vi "190627_FreCTO.vi"() -> ()   [LabVIEW 2019]
uses:
  <vilib>/rvi/interface/nirviReadWriteControl/nirviReadWriteControl.xnode
  <vilib>/rvi/interface/Simulation/niFpgaSimulationCallBeginRW.vi
  <vilib>/rvi/errors/niLvFpgaAdjustHostInterfaceError.vi
  <vilib>/rvi/interface/nirviMethod/nirviMethod.xnode
  <vilib>/FPGAPlugInAG/Dynamic/niLvFpga_Reset_Dynamic.vi
  <vilib>/FPGAPlugInAG/Dynamic/niLvFpga_Run_Dynamic.vi
  <vilib>/rvi/interface/nirviCloseFPGA/nirviCloseFPGA.xnode
  <vilib>/Platform/TimedLoop/XDataNode/XDataNode.xnode
  <vilib>/Platform/TimedLoop/XDataNode/nitl_modes.ctl
  <vilib>/Platform/TimedLoop/XDataNode/XDNodeRunTimeDep.lvlib
  <vilib>/Platform/TimedLoop/XDataNode/wakeup.ctl
  <vilib>/Platform/TimedLoop/XDataNode/timing_clust.ctl
  <vilib>/rvi/interface/nirviOpenFPGA/nirviOpenFPGA.xnode
  <vilib>/Utility/Variable/NI_VariableUtilities.lvlib
  FPGA_TwoAxisEncoder_revised.vi
  <vilib>/FPGAPlugInAG/Dynamic/niLvFpga_Close_Dynamic.vi
panel:
  in  "X_Type":string(combo)="Notch15"
  in  "X_pole":string(combo)="4352"
  in  "Z_Type":string(combo)="Notch15"
  in  "Z_pole":string(combo)="4952"
  out "Time Slots (sec)":dbl[](array[numeric])
  out "All times (sec)":dbl
  out "one period  length":i32
  out "one period start time":i32
  in  "HOST Sample Rate (Hz)":i32=1000
  in  "LOAD":bool
  out "(LS) RMS X (one) (um)":dbl format="%0.4f"
  out "(LS) MAX ERROR X (um)":dbl format="%0.4f"
  out "(LS) RMS ERROR X (um)":dbl format="%0.4f"
  out "(En) RMS X (one) (um)":dbl format="%0.4f"
  out "(LS) RMS Z (one) (um)":dbl format="%0.4f"
  out "(LS) MAX ERROR Z (um)":dbl format="%0.4f"
  out "(LS) RMS ERROR Z (um)":dbl format="%0.4f"
  out "CMD X (rpm)":dbl[](graph)
  out "Linear Scale Position X (mm)":dbl[](graph)
  out "Linear Scale Position Z (mm)":dbl[](graph)
  out "(En) RMS Z (one) (um)":dbl format="%0.4f"
  out "CMD Z (rpm)":dbl[](graph)
  out "Position X (mm)":dbl[](graph)
  out "Linear Scale Position Error X (um)":dbl[](graph)
  out "Linear Scale Position Error Z (um)":dbl[](graph)
  out "Delay":i32
  out "(En) MAX ERROR X (um)":dbl format="%0.4f"
  out "(En) RMS ERROR X (um)":dbl format="%0.4f"
  out "Encoder Position Error X (um)":dbl[](graph)
  out "Position Command X (mm)":dbl[](graph)
  out "(En) MAX ERROR Z (um)":dbl format="%0.4f"
  out "(En) RMS ERROR Z (um)":dbl format="%0.4f"
  out "Encoder Position Error Z (um)":dbl[](graph)
  in  "RUN":bool
  in  "CLEAR":bool
  out "V Loop":bool
  out "Length(Response)":i32
  out "Length(Command)":i32
  out "Done":bool
  out "Error Out (FPGA)":errorcluster
  out "Error Out (Host)":errorcluster
  out "Position Z (mm)":dbl[](graph)
  out "FPGA INITIALIZED":bool
  in  "FPGA Sample Rate (Hz)":dbl=100000.0
  out "Position Command Z (mm)":dbl[](graph)
  in  "STOP":bool
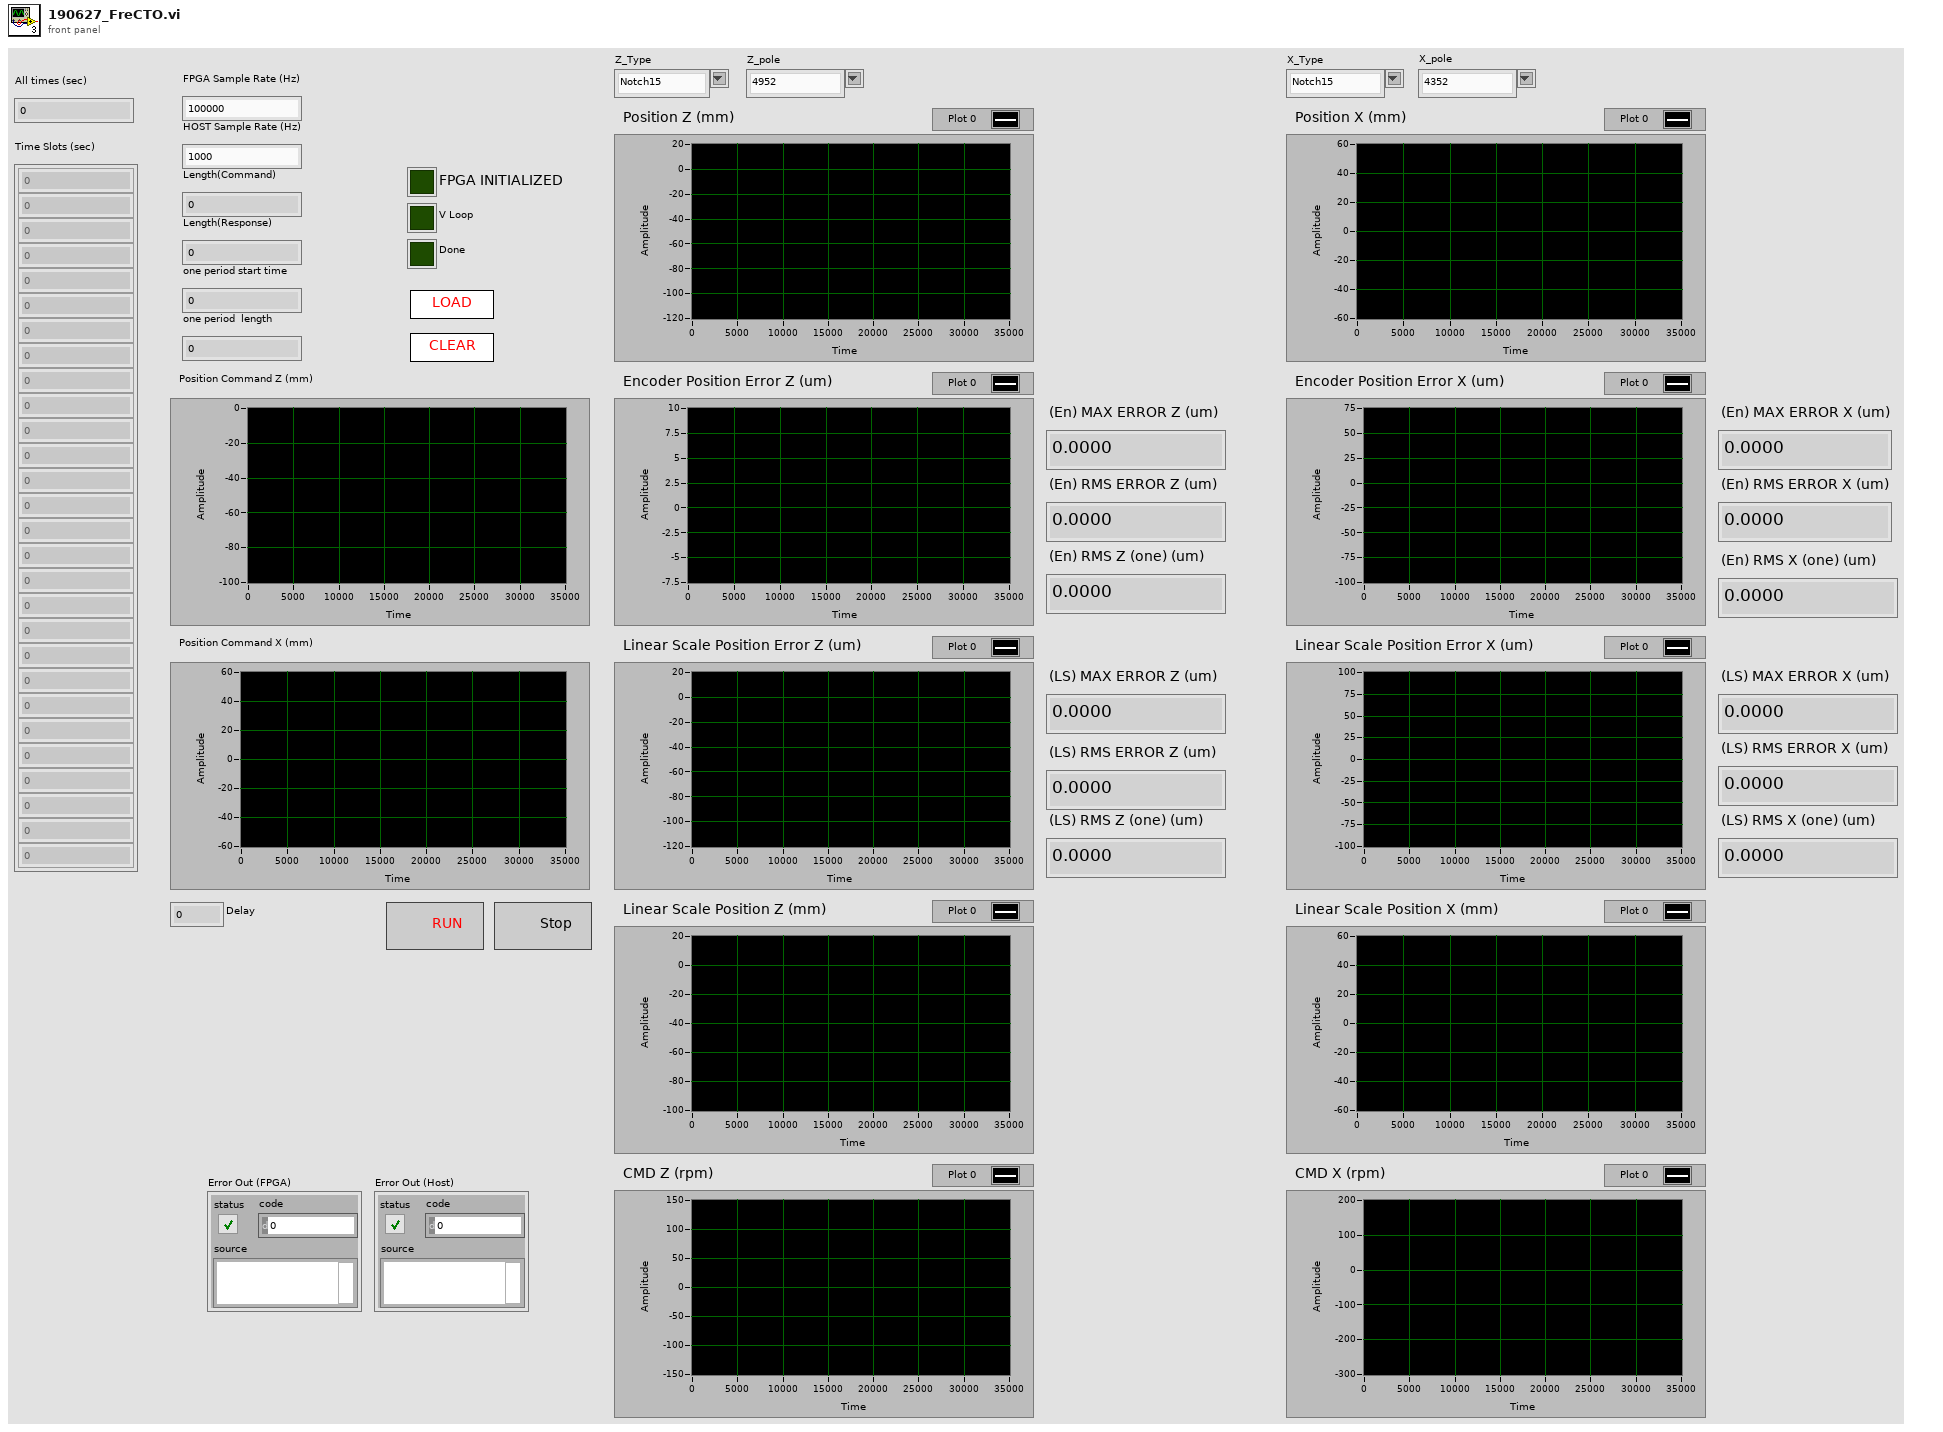
[diagram p1: front panel]
types:
  T1 = typedef "XDNodeRunTimeDep.lvlib/timing_clust.ctl" = cluster{"Expected End [f-1]":u64, "Actual End [f-1]":u64, "Finished Late? [f-1]":bool, "Expected End [i-1]":u64, "Actual End [i-1]":u64, "Finished Late? [i-1]":bool, "Expected Start [i]":u64, "Actual Start [i]":u64, "Expected Start [f]":u64, "Actual Start [f]":u64, "Source Name":string, "Structure Name":string, "Period":i64, "Deadline":i64, "Offset":i64, "Start":i64, "Priority":i32, "Timeout":i32, "Mode":T2, "Wakeup Reason":T3, "Error":errorcluster, "Source Type":string, "Secondary Source Type":string, "Global End Time":u64, "Global Start Time":u64, "Frame Duration":u64, "Iteration Duration":u64, "Assigned CPU":i32, "I/O Scan Engine Mode":u32}
  T2 = typedef "XDNodeRunTimeDep.lvlib/nitl_modes.ctl" = enum32{"No Change", "Process missed periods, maintain original phase", "Discard missed periods, maintain original phase", "Process missed periods, ignore original phase", "Discard missed periods, ignore original phase"}
  T3 = typedef "XDNodeRunTimeDep.lvlib/wakeup.ctl" = enum32{"Normal", "Aborted", "Asynchronous wakeup", "Timing source error", "Timed loop error", "Timeout"}
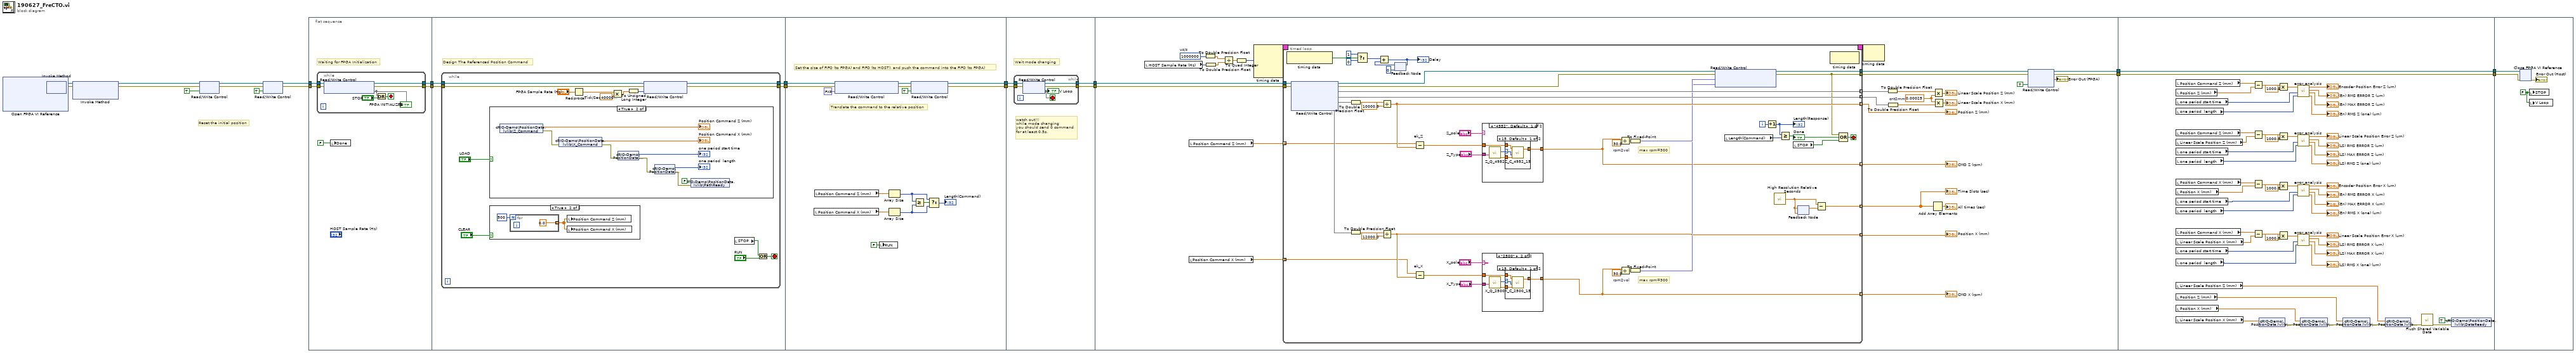
[diagram p0: block diagram]
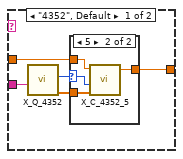
[diagram p4: hidden frame]
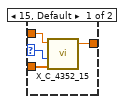
[diagram p5: hidden frame]
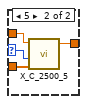
[diagram p6: hidden frame]
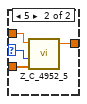
[diagram p7: hidden frame]
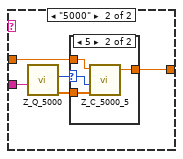
[diagram p8: hidden frame]
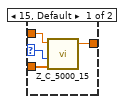
[diagram p9: hidden frame]
diagram:
  # "Reset the initial position"
  n1 = xnode "Open FPGA VI Reference"() -> ("FPGA VI Reference Out"=w7:refnum<k20>, "error out"=w6:errorcluster)  [unwired: 2 in]
  n2 = xnode "Invoke Method"("FPGA VI Reference In"=w7, "error in"=w6) -> ("FPGA VI Reference Out"=w20:refnum<k20>, "error out"=w19:errorcluster)
  n3 = xnode "Invoke Method"("FPGA VI Reference In"=w20, "error in"=w19) -> ("FPGA VI Reference Out"=w5:refnum<k20>, "error out"=w4:errorcluster)  [unwired: 1 in]
  n4 = xnode "Read/Write Control"("FPGA VI Reference In"=w5, "error in"=w4, "Initial"=TRUE ("Reset Encoder")) -> ("FPGA VI Reference Out"=w3:refnum<k20>, "error out"=w2:errorcluster)
  n5 = xnode "Read/Write Control"("FPGA VI Reference In"=w3, "error in"=w2, "Start"=TRUE) -> ("FPGA VI Reference Out"=w14:refnum<k20>, "error out"=w13:errorcluster)
  n6 = flat-sequence {
    tunnel: w14 -> [w29]
    tunnel: w13 -> [w28]
    tunnel: [w27] -> w24
    tunnel: [w26] -> w23
    tunnel: w24 -> [w40]
    tunnel: w23 -> [w39]
    tunnel: [w38] -> w22
    tunnel: [w37] -> w21
    tunnel: w22 -> [w76]
    tunnel: [w79] -> w18
    tunnel: w21 -> [w75]
    tunnel: [w78] -> w16
    tunnel: w18 -> [w83]
    tunnel: [w81] -> w17
    tunnel: w16 -> [w82]
    tunnel: [w80] -> w15
    tunnel: w17 -> [w119]
    tunnel: [w116] -> w11
    tunnel: w15 -> [w118]
    tunnel: [w109] -> w8
    tunnel: w11 -> [w282]
    tunnel: [w282] -> w10
    tunnel: [w281] -> w9
    tunnel: w8 -> [w281]
    tunnel: w10 -> [w285]
    tunnel: w9 -> [w284]
    frame #0 {
      # "Waiting for FPGA Initialization"
      n7 = while {
        tunnel: w29 -> [w36]
        tunnel: w28 -> [w33]
        tunnel: [w32] -> w26
        tunnel: [w31] -> w27
        stop <- w35 stop-if-true
        n8 = xnode "Read/Write Control"("FPGA VI Reference In"=w36, "error in"=w33) -> ("FPGA VI Reference Out"=w31:refnum<k20>, "error out"=w32:errorcluster, "SYSTEM INITIALIZED"=w30)
        "FPGA INITIALIZED" <- w30
        n9 = Or(x=w30, y="STOP") -> (x .or. y?=w35:bool)
      }
      n10 = local write "Done"(FALSE ("Done")) -> ()
    }
    frame #1 {
      # "Design The Referenced Position Command"
      n11 = while {
        tunnel: w40 -> [w54]
        tunnel: w39 -> [w53]
        tunnel: [w48] -> w38
        tunnel: [w47] -> w37
        stop <- w46 stop-if-true
        w50 = 40000000.0  # Tick/Sec
        n12 = case shown="True" "LOAD" {
          frame False {
          }
          frame True {
            n13 = shared-variable "cRIO-Demo\\PositionData.lvlib\\Z_Command"() -> (→"Position Command Z (mm)":dbl[], error out=w65:errorcluster)  [unwired: 1 in]
            n14 = shared-variable "cRIO-Demo\\PositionData.lvlib\\X_Command"(error in=w65) -> (→"Position Command X (mm)":dbl[], error out=w61:errorcluster)
            n15 = shared-variable "cRIO-Demo\\PositionData.lvlib\\t0"(error in=w61) -> (→"one period start time":i32, error out=w62:errorcluster)
            n16 = shared-variable "cRIO-Demo\\PositionData.lvlib\\tL"(error in=w62) -> (→"one period  length":i32, error out=w60:errorcluster)
            n17 = shared-variable "cRIO-Demo\\PositionData.lvlib\\PathReady"(FALSE ("PathReady"), error in=w60) -> ()  [unwired: 1 out]
          }
        }
        n18 = case shown="True" "CLEAR" {
          frame False {
          }
          frame True {
            n19 = for {
              N: 500 -> [_]
              tunnel: [0.0 ("element")] -> w56 mode=indexing
            }
            n20 = local write "Position Command Z (mm)"(w56) -> ()
            n21 = local write "Position Command X (mm)"(w56) -> ()
          }
        }
        n22 = Reciprocal(x="FPGA Sample Rate (Hz)") -> (1/x=w51:dbl)
        n23 = Multiply(x=w51, y=w50) -> (x*y=w52:dbl)
        n24 = To Unsigned Long Integer(number=w52) -> (unsigned 32bit integer=w49:u32)
        n25 = xnode "Read/Write Control"("FPGA VI Reference In"=w54, "error in"=w53, "Loop Delay (Tick)"=w49) -> ("FPGA VI Reference Out"=w48:refnum<k20>, "error out"=w47:errorcluster)
        n26 = local read "STOP"() -> (w45:bool)
        n27 = Or(x=w45, y="RUN") -> (x .or. y?=w46:bool)
      }
    }
    frame #2 {
      # "Translate the command to the relative position"
      # "Set the size of FIFO (to FPGA) and FIFO (to HOST), and push the command into the FIFO (to FPGA)"
      n28 = local read "Position Command X (mm)"() -> (w67:dbl[])
      n29 = local read "Position Command Z (mm)"() -> (w68:dbl[])
      n30 = xnode "Read/Write Control"("FPGA VI Reference In"=w76, "Output Votage Bound (vol)"=fxp<+,20,5> 10.0) -> ()  [unwired: 1 in, 2 out]
      n31 = local write "RUN"(FALSE) -> ()
      n32 = Array Size(array=w68) -> (size(s)=w71:i32)
      n33 = Array Size(array=w67) -> (size(s)=w70:i32)
      n34 = xnode "Read/Write Control"("FPGA VI Reference In"=w76, "error in"=w75, "HOST READY?"=TRUE) -> ("FPGA VI Reference Out"=w79:refnum<k20>, "error out"=w78:errorcluster)
      n35 = Greater Or Equal?(x=w71, y=w70) -> (x >= y?=w72:bool)
      n36 = Select(t=w71, s=w72, f=w70) -> (s? t:f=→"Length(Command)":i32)
    }
    frame #3 {
      # "watch out!!!\nwhile mode changing\nyou should send 0 command\nfor at least 0.5s."
      # "Wait mode changing"
      n37 = while {
        tunnel: w83 -> [w88]
        tunnel: w82 -> [w87]
        tunnel: [w86] -> w81
        tunnel: [w85] -> w80
        stop <- w84 stop-if-true
        n38 = xnode "Read/Write Control"("FPGA VI Reference In"=w88, "error in"=w87) -> ("FPGA VI Reference Out"=w86:refnum<k20>, "error out"=w85:errorcluster, "V Loop"=w84)
        "V Loop" <- w84
      }
    }
    frame #4 {
      w91 = 0.00025  # cnt2mm
      w113 = 1000000  # us/s
      n39 = local read "HOST Sample Rate (Hz)"() -> (w102:i32)
      n40 = local read "Position Command X (mm)"() -> (w100:dbl[])
      n41 = local read "Position Command Z (mm)"() -> (w101:dbl[])
      n42 = To Double Precision Float(number=w113) -> (double precision float=w105:dbl)
      n43 = To Double Precision Float(number=w102) -> (double precision float=w106:dbl)
      n44 = Divide(x=w105, y=w106) -> (x/y=w112:dbl)
      n45 = To Quad Integer(1:w112) -> (0:w111:i64)
      n46 = node-c288(w111) -> (w115:T1)  [unwired: 3 in]
      n47 = timed-loop {
        tunnel: w119 -> [w151]
        tunnel: w118 -> [w149]
        tunnel: [w135] -> w117
        timing: w115 -> [_]
        timing-out: [_] -> w114
        tunnel: [w134] -> w110
        tunnel: [w145] -> w96 mode=indexing
        tunnel: [w142] -> w94 mode=indexing
        tunnel: [w120] -> w103 mode=indexing
        tunnel: [w146] -> w95 mode=indexing
        tunnel: w101 -> [w129] mode=indexing
        tunnel: w100 -> [w128] mode=indexing
        tunnel: [w121] -> w99 mode=indexing
        tunnel: [w140] -> w93 mode=indexing
        tunnel: [w130] -> w89 mode=indexing
        i -> [w162]
        stop <- w167 stop-if-true
        w144 = 30.0  # rpm2vol
        w163 = 30.0  # rpm2vol
        # "max rpm=300"
        # "max rpm=300"
        n48 = node-c288() -> (w156:bool)  [unwired: 1 in]
        n49 = xnode "Read/Write Control"("FPGA VI Reference In"=w151, "error in"=w149) -> ("FPGA VI Reference Out"=w139:refnum<k20>, "error out"=w138:errorcluster, "Line Scale Z (count)"=w142, "Line Scale X (count)"=w140, "Encoder Z (count)"=w141, "Encoder X (count)"=w133)
        n50 = To Double Precision Float(number=w141) -> (double precision float=w161:dbl)
        n51 = To Double Precision Float(number=w133) -> (double precision float=w148:dbl)
        n52 = Select(t=1, s=w156, f=0) -> (s? t:f=w155:i32)
        n53 = Divide(x=w161, y=10000.0) -> (x/y=w145:dbl)
        n54 = Divide(x=w148, y=12000.0) -> (x/y=w146:dbl)
        n55 = feedback #1(0) -> (w153:i32)
        n56 = Add(x=w155, y=w153) -> (x+y=w154:i32)
        "Delay" <- w154
        n57 = feedback-in #1(w154) -> ()
        n58 = Subtract "ek_Z"(x=w129, y=w145) -> (x-y=w125:dbl)
        n59 = Subtract "ek_X"(x=w128, y=w146) -> (x-y=w122:dbl)
        n60 = case shown="\"4952\", Default" "Z_pole" {
          tunnel: "Z_Type" -> [w198 w211]
          tunnel: w125 -> [w195 w208]
          tunnel: [w194 w207] -> w120
          frame "4952", Default {
            n61 = call "Z_Q_4952.vi"("Type"=w198) -> ("Qn"=w196:dbl[], "L"=w197:i32)  [unwired: 9 in]
            n62 = case shown="15, Default" w197 {
              selector: w197 -> [w200 w204]
              tunnel: w196 -> [w199 w203]
              tunnel: w195 -> [w202 w206]
              tunnel: [w201 w205] -> w194
              frame 15, Default {
                n63 = call "Z_C_4952_15.vi"("ek"=w202, "length"=w200, "q"=w199) -> ("uk"=w201:dbl)  [unwired: 4 in]
              }
              frame 5 {
                n64 = call "Z_C_4952_5.vi"("ek"=w206, "length"=w204, "q"=w203) -> ("uk"=w205:dbl)  [unwired: 4 in]
              }
            }
          }
          frame "5000" {
            n65 = call "Z_Q_5000.vi"("Type"=w211) -> ("Qn"=w209:dbl[], "L"=w210:i32)  [unwired: 9 in]
            n66 = case shown="5" w210 {
              selector: w210 -> [w213 w217]
              tunnel: w209 -> [w212 w216]
              tunnel: w208 -> [w215 w219]
              tunnel: [w214 w218] -> w207
              frame 15, Default {
                n67 = call "Z_C_5000_15.vi"("ek"=w215, "length"=w213, "q"=w212) -> ("uk"=w214:dbl)  [unwired: 4 in]
              }
              frame 5 {
                n68 = call "Z_C_5000_5.vi"("ek"=w219, "length"=w217, "q"=w216) -> ("uk"=w218:dbl)  [unwired: 4 in]
              }
            }
          }
        }
        n69 = case shown="\"2500\"" "X_pole" {
          tunnel: "X_Type" -> [w172 w185]
          tunnel: w122 -> [w169 w182]
          tunnel: [w168 w181] -> w121
          frame "4352", Default {
            n70 = call "X_Q_4352.vi"("Type"=w172) -> ("Qn"=w170:dbl[], "L"=w171:i32)  [unwired: 9 in]
            n71 = case shown="5" w171 {
              selector: w171 -> [w174 w178]
              tunnel: w170 -> [w173 w177]
              tunnel: w169 -> [w176 w180]
              tunnel: [w175 w179] -> w168
              frame 15, Default {
                n72 = call "X_C_4352_15.vi"("ek"=w176, "length"=w174, "q"=w173) -> ("uk"=w175:dbl)  [unwired: 4 in]
              }
              frame 5 {
                n73 = call "X_C_4352_5.vi"("ek"=w180, "length"=w178, "q"=w177) -> ("uk"=w179:dbl)  [unwired: 4 in]
              }
            }
          }
          frame "2500" {
            n74 = call "X_Q_2500.vi"("Type"=w185) -> ("Qn"=w183:dbl[], "L"=w184:i32)  [unwired: 9 in]
            n75 = case shown="15, Default" w184 {
              selector: w184 -> [w187 w191]
              tunnel: w183 -> [w186 w190]
              tunnel: w182 -> [w189 w193]
              tunnel: [w188 w192] -> w181
              frame 15, Default {
                n76 = call "X_C_2500_15.vi"("ek"=w189, "length"=w187, "q"=w186) -> ("uk"=w188:dbl)  [unwired: 4 in]
              }
              frame 5 {
                n77 = call "X_C_2500_5.vi"("ek"=w193, "length"=w191, "q"=w190) -> ("uk"=w192:dbl)  [unwired: 4 in]
              }
            }
          }
        }
        n78 = Divide(x=w120, y=w163) -> (x/y=w164:fxp<+/-,20,5>)
        n79 = Divide(x=w121, y=w144) -> (x/y=w143:fxp<+/-,20,5>)
        n80 = To Fixed-Point(number=w164) -> (fixed-point=w137:fxp<+/-,20,5>)  [unwired: 1 in]
        n81 = To Fixed-Point(number=w143) -> (fixed-point=w136:fxp<+/-,20,5>)  [unwired: 1 in]
        n82 = xnode "Read/Write Control"("FPGA VI Reference In"=w139, "error in"=w138, "Velocity Command Z (vol)"=w137, "Velocity Command X (vol)"=w136) -> ("FPGA VI Reference Out"=w135:refnum<k20>, "error out"=w134:errorcluster)
        n83 = local read "Length(Command)"() -> (w150:i32)
        n84 = Increment(x=w162) -> (x+1=w159:i32)
        "Length(Response)" <- w159
        n85 = call <vilib>:"High Resolution Relative Seconds.vi"() -> ("relative seconds"=w132:dbl)
        n86 = Greater Or Equal?(x=w159, y=w150) -> (x >= y?=w166:bool)
        "Done" <- w166
        n87 = local read "STOP"() -> (w165:bool)
        n88 = feedback #2(w132) -> (w131:dbl)
        n89 = feedback-in #2(w132) -> ()
        n90 = Subtract(x=w132, y=w131) -> (x-y=w130:dbl)
        n91 = node-c288() -> ()  [unwired: 1 in, 1 out]
        n92 = Compound Arithmetic op=OR(w134, w166, w165) -> (w167:bool)
      }
      "Position Z (mm)" <- w96
      "Position X (mm)" <- w95
      "CMD Z (rpm)" <- w103
      "CMD X (rpm)" <- w99
      "Time Slots (sec)" <- w89
      n93 = node-c288(w114) -> ()  [unwired: 1 out]
      n94 = To Double Precision Float(number=w94) -> (double precision float=w92:dbl[])
      n95 = To Double Precision Float(number=w93) -> (double precision float=w98:dbl[])
      n96 = Add Array Elements(numeric array=w89) -> (sum=→"All times (sec)":dbl)
      n97 = Multiply(x=w92, y=w91) -> (x*y=→"Linear Scale Position Z (mm)":dbl[])
      n98 = Multiply(x=w91, y=w98) -> (x*y=→"Linear Scale Position X (mm)":dbl[])
      n99 = xnode "Read/Write Control"("FPGA VI Reference In"=w117, "error in"=w110, "stop"=TRUE) -> ("FPGA VI Reference Out"=w116:refnum<k20>, "error out"=w109:errorcluster, "Error Out"=→"Error Out (FPGA)")
    }
    frame #5 {
      n100 = local read "Position Command Z (mm)"() -> (w280:dbl[])
      n101 = local read "Position Z (mm)"() -> (w279:dbl[])
      n102 = local read "one period start time"() -> (w270:i32)
      n103 = local read "one period  length"() -> (w269:i32)
      n104 = local read "Position Command Z (mm)"() -> (w233:dbl[])
      n105 = local read "Linear Scale Position Z (mm)"() -> (w276:dbl[])
      n106 = local read "one period start time"() -> (w264:i32)
      n107 = local read "one period  length"() -> (w263:i32)
      n108 = local read "Position Command X (mm)"() -> (w251:dbl[])
      n109 = local read "Position X (mm)"() -> (w250:dbl[])
      n110 = local read "one period start time"() -> (w249:i32)
      n111 = local read "one period  length"() -> (w248:i32)
      n112 = local read "Position Command X (mm)"() -> (w234:dbl[])
      n113 = local read "Linear Scale Position X (mm)"() -> (w247:dbl[])
      n114 = local read "one period start time"() -> (w246:i32)
      n115 = local read "one period  length"() -> (w245:i32)
      n116 = local read "Linear Scale Position Z (mm)"() -> (w243:dbl[])
      n117 = local read "Position Z (mm)"() -> (w235:dbl[])
      n118 = local read "Position X (mm)"() -> (w236:dbl[])
      n119 = local read "Linear Scale Position X (mm)"() -> (w244:dbl[])
      n120 = Subtract(x=w280, y=w279) -> (x-y=w277:dbl[])
      n121 = Subtract(x=w233, y=w276) -> (x-y=w228:dbl[])
      n122 = Subtract(x=w251, y=w250) -> (x-y=w261:dbl[])
      n123 = Subtract(x=w234, y=w247) -> (x-y=w232:dbl[])
      n124 = shared-variable "cRIO-Demo\\PositionData.lvlib\\X_LS"(w244) -> (error out=w242:errorcluster)  [unwired: 1 in]
      n125 = Multiply(x=w277, y=1000.0) -> (x*y=w275:dbl[])
      n126 = Multiply(x=w228, y=1000.0) -> (x*y=w227:dbl[])
      n127 = Multiply(x=w261, y=1000.0) -> (x*y=w262:dbl[])
      n128 = Multiply(x=w232, y=1000.0) -> (x*y=w230:dbl[])
      n129 = call "error_analysis.vi"("tLength"=w269, "t0"=w270, "data in (um)"=w275) -> ("rms (one) (um)"=→"(En) RMS Z (one) (um)":dbl, "max err (um)"=→"(En) MAX ERROR Z (um)":dbl, "rms (all) (um)"=→"(En) RMS ERROR Z (um)":dbl, "data out (um)"=→"Encoder Position Error Z (um)":dbl[])  [unwired: 5 in]
      n130 = call "error_analysis.vi"("tLength"=w263, "t0"=w264, "data in (um)"=w227) -> ("rms (one) (um)"=→"(LS) RMS Z (one) (um)":dbl, "max err (um)"=→"(LS) MAX ERROR Z (um)":dbl, "rms (all) (um)"=→"(LS) RMS ERROR Z (um)":dbl, "data out (um)"=→"Linear Scale Position Error Z (um)":dbl[])  [unwired: 5 in]
      n131 = call "error_analysis.vi"("tLength"=w248, "t0"=w249, "data in (um)"=w262) -> ("rms (one) (um)"=→"(En) RMS X (one) (um)":dbl, "max err (um)"=→"(En) MAX ERROR X (um)":dbl, "rms (all) (um)"=→"(En) RMS ERROR X (um)":dbl, "data out (um)"=→"Encoder Position Error X (um)":dbl[])  [unwired: 5 in]
      n132 = call "error_analysis.vi"("tLength"=w245, "t0"=w246, "data in (um)"=w230) -> ("rms (one) (um)"=→"(LS) RMS X (one) (um)":dbl, "max err (um)"=→"(LS) MAX ERROR X (um)":dbl, "rms (all) (um)"=→"(LS) RMS ERROR X (um)":dbl, "data out (um)"=→"Linear Scale Position Error X (um)":dbl[])  [unwired: 5 in]
      n133 = shared-variable "cRIO-Demo\\PositionData.lvlib\\X_EN"(w236, error in=w242) -> (error out=w241:errorcluster)
      n134 = shared-variable "cRIO-Demo\\PositionData.lvlib\\Z_EN"(w235, error in=w241) -> (error out=w240:errorcluster)
      n135 = shared-variable "cRIO-Demo\\PositionData.lvlib\\Z_LS"(w243, error in=w240) -> (error out=w239:errorcluster)
      n136 = call <vilib>:"Flush Shared Variable Data.vi"("error in (no error)"=w239) -> ("error out"=w238:errorcluster)  [unwired: 10 in]
      n137 = shared-variable "cRIO-Demo\\PositionData.lvlib\\DataReady"(TRUE, error in=w238) -> ()  [unwired: 1 out]
    }
    frame #6 {
      w283 = FALSE ("STOP")
      n138 = xnode "Close FPGA VI Reference"("FPGA VI Reference In"=w285, "error in"=w284) -> ("error out"=→"Error Out (Host)":errorcluster)
      n139 = local write "STOP"(w283) -> ()
      n140 = local write "V Loop"(w283) -> ()
    }
  }
